vi "LSX Move Rel TVRO.vi"(5 "bWait":i32, 6 "dR":dbl, 7 "dZ":dbl, 8 "error in (no error)":errorcluster, 9 "dY":dbl, 10 "dX":dbl, 11 "lLSID":i32) -> (0 "error out":errorcluster, 3 "function return":i32)   [LabVIEW 2018, in "Tango.lvlib"]
doc: "TANGOAPI int TANGOCALL LSX_MoveRelTVRO (int lLSID, double dX, double dY, double dZ, double dR, BOOL bWait);"
uses:
  Tango.lvlib
  SubVIs/Tango_DLL.dll
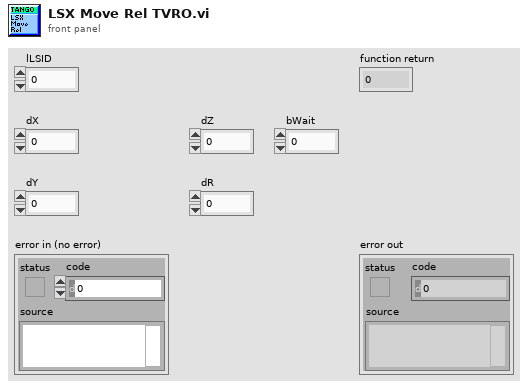
[diagram p1: front panel]
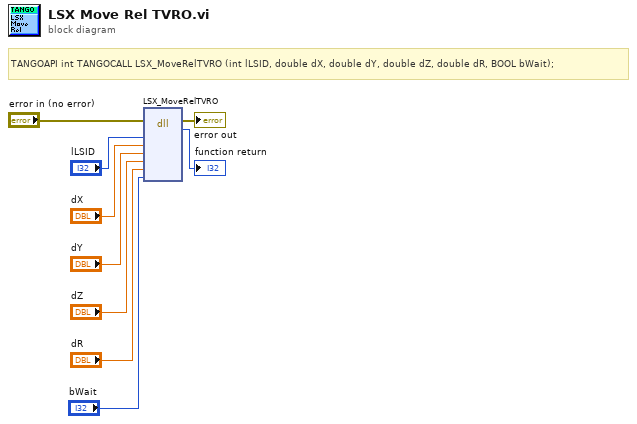
[diagram p0: block diagram]
diagram:
  # "TANGOAPI int TANGOCALL LSX_MoveRelTVRO (int lLSID, double dX, double dY, double dZ, double dR, BOOL bWait);"
  n1 = dll-call lib="C:/Users/Familie/Documents/LabviewIX81/lib/TANGO Stage/SubVIs/Tango_DLL.*" fn="LSX_MoveRelTVRO"(error in="error in (no error)", "lLSID"="lLSID", "dX"="dX", "dY"="dY", "dZ"="dZ", "dR"="dR", "bWait"="bWait") -> (error out=→"error out":errorcluster, →"function return":i32)  [unwired: 8 in, 1 out]
